vi "Event-Driven State Machine - VI Window Customization.vi"() -> ()   [LabVIEW 2020]
uses:
  support/State Machine Data.ctl
  support/States.ctl
  <vilib>/DAQmx/miscellaneous.llb/DAQmx Fill In Error Info.vi
  <vilib>/DAQmx/read.llb/DAQmx Read (Analog 2D DBL NChan NSamp).vi
  <vilib>/DAQmx/write.llb/DAQmx Write (Analog DBL 1Chan 1Samp).vi
  <vilib>/DAQmx/create/channels.llb/DAQmx Create Channel (AI-Voltage-Basic).vi
  <vilib>/DAQmx/configure/timing.llb/DAQmx Timing (Sample Clock).vi
  <vilib>/DAQmx/create/channels.llb/DAQmx Create Channel (AO-Voltage-Basic).vi
  <vilib>/Utility/file.llb/Write Delimited Spreadsheet (DBL).vi
panel:
  out "RMS Results Per Channel":dbl[](array[numeric])
  out "Threshold exceeded?":bool
  in  "Acquire":bool
  in  "Samples per channel":i32=100
  in  "Sample Rate":dbl=1000.0
  in  "AI Voltage Channel":tag="PCI-6221/ai0, PCI-6221/ai2:3"
  in  "AO Voltage Channel":tag="PCI-6221/ao0"
  in  "Generate Stimulus":bool
  in  "Threshold (rms)":dbl=1.0
  in  "Clear":bool
  in  "Exit":bool
  out "Graph":dbl[][](graph)
  # "Analysis"
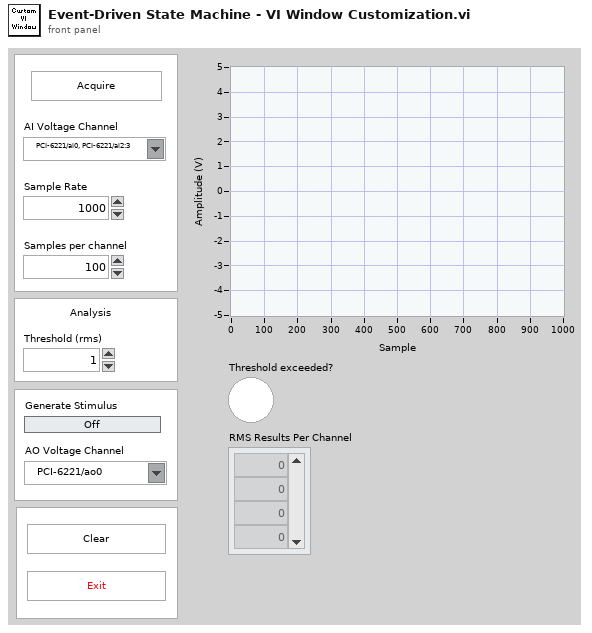
[diagram p1: front panel]
types:
  T1 = enum16{"Always On", "Always Off", "Off While Running"}
  T2 = typedef "States.ctl" = enum16{"Initialize", "Wait for Event", "Acquire", "Analyze", "Log", "Clear", "Update Stimulus", "Update UI", "Exit"}
  T3 = typedef "State Machine Data.ctl" = cluster{"Acquisition Data":dbl[][], "Stimulus Value":bool}
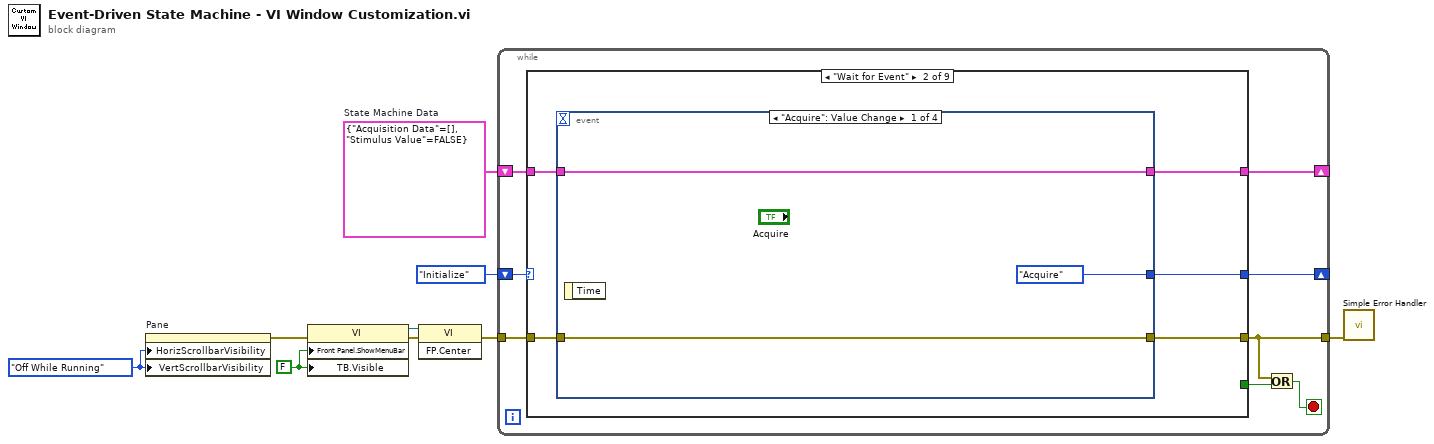
[diagram p0: block diagram]
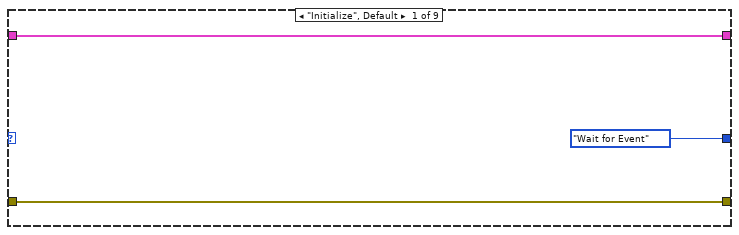
[diagram p2: hidden frame]
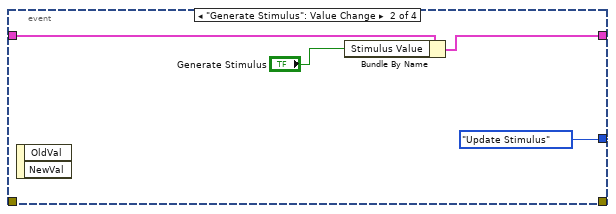
[diagram p3: hidden frame]
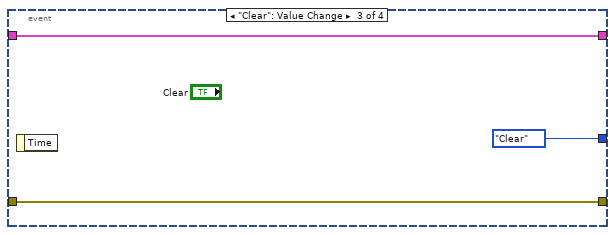
[diagram p4: hidden frame]
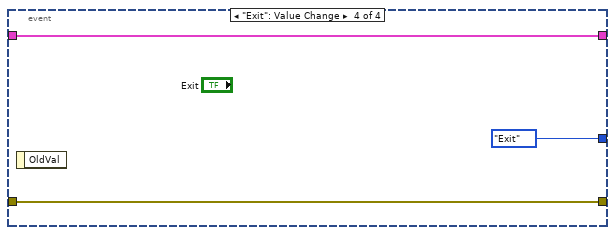
[diagram p5: hidden frame]
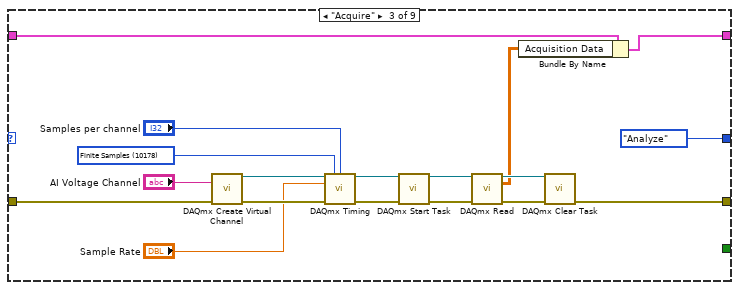
[diagram p6: hidden frame]
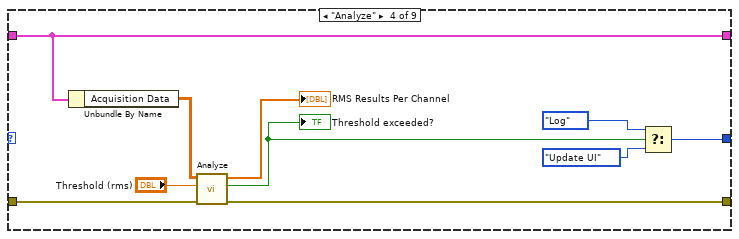
[diagram p7: hidden frame]
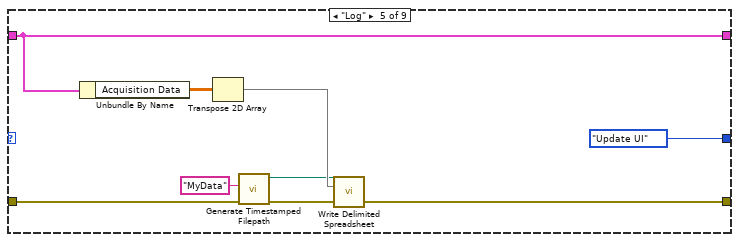
[diagram p8: hidden frame]
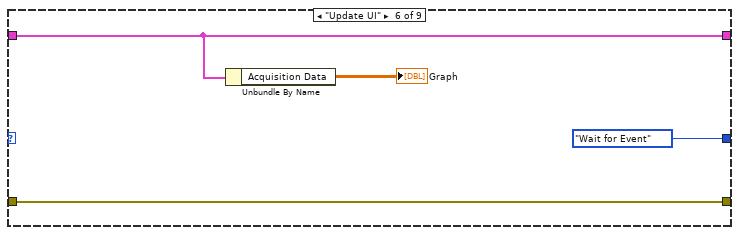
[diagram p9: hidden frame]
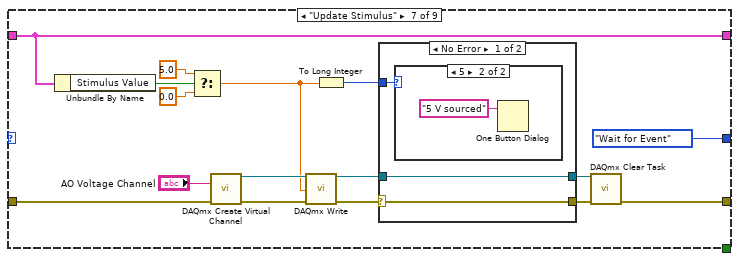
[diagram p10: hidden frame]
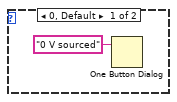
[diagram p11: hidden frame]
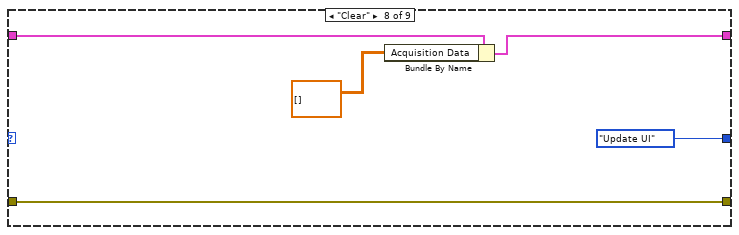
[diagram p13: hidden frame]
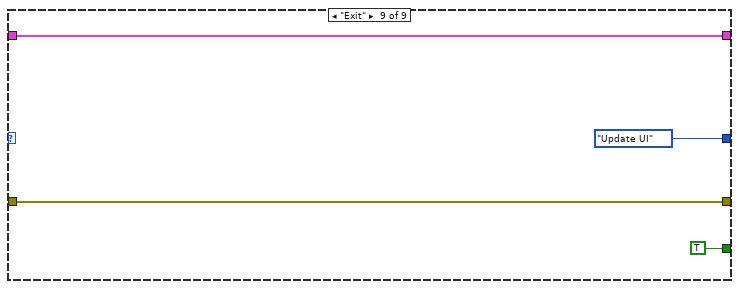
[diagram p14: hidden frame]
diagram:
  w4 = FALSE
  w6 = T1."Off While Running" ("Horizontal Scrollbar Visibility")
  w8 = T3 {"Acquisition Data"=[], "Stimulus Value"=FALSE}  # State Machine Data
  n1 = property on="Pane" class="Pane"("HorizScrollbarVisibility"=w6, "VertScrollbarVisibility"=w6) -> (error out=w5:errorcluster)  [unwired: 2 in, 1 out]
  n2 = property class="VI"(error in=w5, "Front Panel.ShowMenuBar"=w4, "TB.Visible"=w4) -> (reference out=w3:refnum<vi>, error out=w2:errorcluster)  [unwired: 1 in]
  n3 = invoke class="VI" method="FP.Center"(reference=w3, error in=w2) -> (error out=w1:errorcluster)  [unwired: 1 in, 2 out]
  n4 = while {
    shift-right: [w14] -> _
    shift-left: States."Initialize" ("States") -> [w17]
    shift-right: [w15] -> _
    shift-left: w8 -> [w16]
    tunnel: w1 -> [w13]
    tunnel: [w12] -> w7
    stop <- w10 stop-if-true
    n5 = case shown="\"Wait for Event\"" w17 {
      tunnel: w16 -> [w20 w25 w44 w66 w74 w78 w95 w106 w110]
      tunnel: [w20 w24 w40 w66 w74 w78 w95 w104 w110] -> w15
      tunnel: [States."Wait for Event" ("States") w21 States."Analyze" ("States") w58 States."Update UI" ("States") States."Wait for Event" ("States") States."Wait for Event" ("States") States."Update UI" ("States") States."Update UI" ("States")] -> w14
      tunnel: w13 -> [w18 w23 w56 w63 w72 w79 w89 w107 w111]
      tunnel: [w18 w22 w42 w61 w68 w79 w90 w107 w111] -> w12
      tunnel: [_ _ _ _ _ _ _ _ TRUE] -> w11
      frame "Initialize", Default {
      }
      frame "Wait for Event" {
        n6 = event shown="[0] \"Acquire\": Value Change" {
          selector: _ -> [_ _ _ _]
          dyn-events: _ -> [_ _ _ _]
          timeout: _ -> [_ _ _ _]
          tunnel: w25 -> [w27 w32 w35 w37]
          tunnel: [w27 w31 w35 w37] -> w24
          tunnel: w23 -> [w28 _ w34 w38]
          tunnel: [w28 _ w34 w38] -> w22
          tunnel: [States."Acquire" ("Enum") States."Update Stimulus" ("Enum") States."Clear" ("Enum") States."Exit" ("Enum")] -> w21
          event "Acquire": Value Change {
            n7 = event-data() -> ()  [unwired: 1 in, 1 out]
          }
          event "Generate Stimulus": Value Change {
            n8 = event-data() -> ()  [unwired: 1 in, 2 out]
            n9 = Bundle By Name(cluster=w32, "Stimulus Value"="Generate Stimulus") -> (w31:T3)
          }
          event "Clear": Value Change {
            n10 = event-data() -> ()  [unwired: 1 in, 1 out]
          }
          event "Exit": Value Change {
            n11 = event-data() -> ()  [unwired: 1 in, 1 out]
          }
        }
      }
      frame "Acquire" {
        w52 = 10178 items=["Finite Samples"=10178, "Continuous Samples"=10123, "Hardware Timed Single Point"=12522] ("sample mode")
        n12 = call-poly <vilib>:"DAQmx Create Virtual Channel.vi"("physical channels"="AI Voltage Channel", "error in"=w56) -> ("task out"=w53:refnum<k21>, "error out"=w54:errorcluster)  [unwired: 12 in]
        n13 = call-poly <vilib>:"DAQmx Timing.vi"("task/channels in"=w53, "sample mode"=w52, "samples per channel"="Samples per channel", "rate"="Sample Rate", "error in"=w54) -> ("task out"=w50:refnum<k21>, "error out"=w49:errorcluster)  [unwired: 9 in]
        n14 = call <vilib>:"DAQmx Start Task.vi"("task/channels in"=w50, "error in"=w49) -> ("task out"=w48:refnum<k21>, "error out"=w47:errorcluster)  [unwired: 12 in]
        n15 = call-poly <vilib>:"DAQmx Read.vi"("task/channels in"=w48, "error in"=w47) -> ("task out"=w46:refnum<k21>, "data"=w43:dbl[][], "error out"=w45:errorcluster)  [unwired: 11 in]
        n16 = Bundle By Name(cluster=w44, "Acquisition Data"=w43) -> (w40:T3)
        n17 = call <vilib>:"DAQmx Clear Task.vi"("task in"=w46, "error in"=w45) -> ("error out"=w42:errorcluster)  [unwired: 13 in]
      }
      frame "Analyze" {
        n18 = Unbundle By Name(w66) -> ("Acquisition Data"=w65:dbl[][])
        n19 = call "Analyze.vi"("error in (no error)"=w63, "Threshold (rms)"="Threshold (rms)", "N-Channel Data (2D DBL)"=w65) -> ("error out"=w61:errorcluster, "Threshold Exceeded?"=w57:bool, "N-Channel RMS Results"=→"RMS Results Per Channel":dbl[])  [unwired: 5 in, 1 out]
        "Threshold exceeded?" <- w57
        n20 = Select(t=States."Log" ("States"), s=w57, f=States."Update UI" ("States")) -> (s? t:f=w58:T2)
      }
      frame "Log" {
        n21 = Unbundle By Name(w74) -> ("Acquisition Data"=w75:dbl[][])
        n22 = Transpose 2D Array(2D array=w75) -> (transposed array=w71:dbl[][])
        n23 = call "Generate Timestamped Filepath.vi"("Error In"=w72, "appended filename"="MyData") -> ("Error Out"=w69:errorcluster, "timestamped relative filepath"=w70:path)  [unwired: 8 in]
        n24 = call-poly <vilib>:"Write Delimited Spreadsheet.vi"("file path (dialog if empty)"=w70, "2D data"=w71, "error in (no error)"=w69) -> ("error out"=w68:errorcluster)  [unwired: 11 in, 1 out]
      }
      frame "Update UI" {
        n25 = Unbundle By Name(w78) -> ("Acquisition Data"=→"Graph":dbl[][])
      }
      frame "Update Stimulus" {
        n26 = Unbundle By Name(w95) -> ("Stimulus Value"=w86:bool)
        n27 = Select(t=5.0, s=w86, f=0.0) -> (s? t:f=w85:dbl)
        n28 = call-poly <vilib>:"DAQmx Create Virtual Channel.vi"("physical channels"="AO Voltage Channel", "error in"=w89) -> ("task out"=w92:refnum<k21>, "error out"=w91:errorcluster)  [unwired: 12 in]
        n29 = call-poly <vilib>:"DAQmx Write.vi"("task/channels in"=w92, "data"=w85, "error in"=w91) -> ("task out"=w82:refnum<k21>, "error out"=w83:errorcluster)  [unwired: 10 in, 1 out]
        n30 = To Long Integer(number=w85) -> (32bit integer=w84:i32)
        n31 = case shown="No Error" w83 {
          selector: w83 -> [w96 w101]
          tunnel: w84 -> [w98 _]
          tunnel: w82 -> [w97 w102]
          tunnel: [w97 w102] -> w81
          tunnel: [w96 w101] -> w80
          frame No Error {
            n32 = case shown="5" w98 {
              frame 0, Default {
                n33 = One Button Dialog(message="0 V sourced") -> ()  [unwired: 1 in, 1 out]
              }
              frame 5 {
                n34 = One Button Dialog(message="5 V sourced") -> ()  [unwired: 1 in, 1 out]
              }
            }
          }
          frame Error {
          }
        }
        n35 = call <vilib>:"DAQmx Clear Task.vi"("task in"=w81, "error in"=w80) -> ("error out"=w90:errorcluster)  [unwired: 13 in]
      }
      frame "Clear" {
        n36 = Bundle By Name(cluster=w106, "Acquisition Data"=dbl[][] []) -> (w104:T3)
      }
      frame "Exit" {
      }
    }
    n37 = Or(x=w12, y=w11) -> (x .or. y?=w10:bool)
  }
  n38 = call <vilib>:"Simple Error Handler.vi"("error in (no error)"=w7) -> ()  [unwired: 4 in, 5 out]
